vi "Controller_v6.vi"(10 "Sensors":T2) -> (0 "To Target Lossy Data":T1, 3 "Motor Command":dbl)   [LabVIEW 2018]
uses:
  Sensor Data.ctl
  Phase Calculator Feedback Cluster.ctl
  Target Lossy Data.ctl
panel:
  in  "Target Lossy Data":T1
  in  "Phase Calculator Feedback":T3
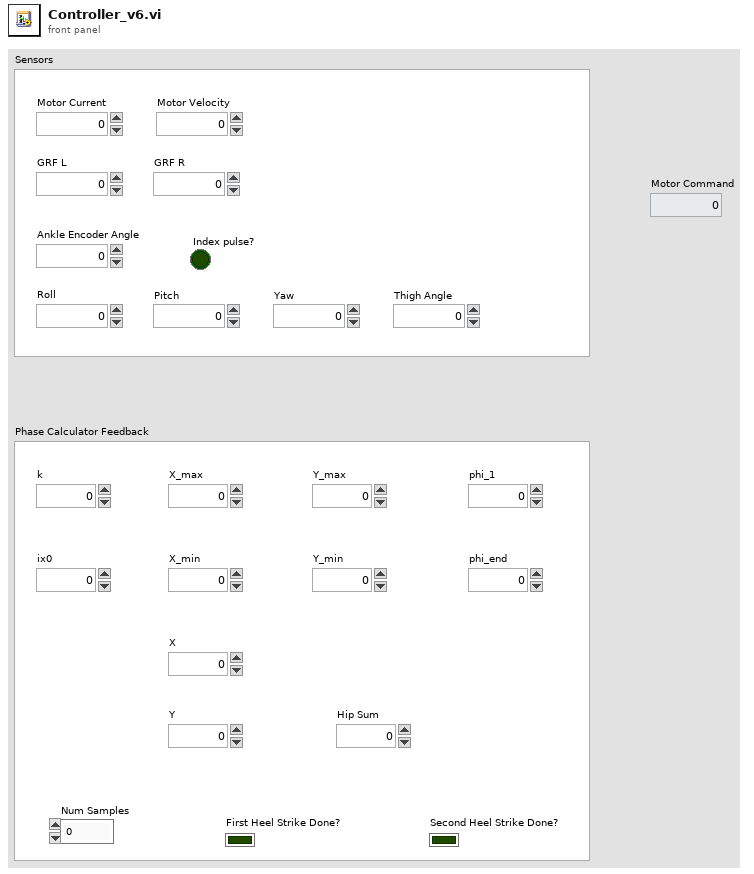
[diagram p1: front panel]
types:
  T1 = typedef "Target Lossy Data.ctl" = cluster{"Active Controller":bool, "Log Trigger":bool, "Sensors":T2, "Motor Command":dbl, "Phase Variable":dbl, "Left HS State":u32, "Left Heel Strike Pulse":bool, "Gait %":dbl, "Torque Reference":dbl, "Passive Torque":dbl, "F_th":dbl, "dF_th":dbl, "d_GRF L":dbl, "GRF L":dbl, "Transmission Ratio":dbl, "Desired Ankle Traj.":dbl, "Right HS State":u32, "Right Heel Strike Pulse":bool, "d_GRF R":dbl, "GRF R":dbl}
  T2 = typedef "Sensor Data.ctl" = cluster{"Motor Current":dbl, "Motor Velocity":dbl, "Ankle Encoder Angle":dbl, "GRF L":dbl, "GRF R":dbl, "Index pulse?":bool, "Roll":dbl, "Pitch":dbl, "Yaw":dbl, "Thigh Angle":dbl}
  T3 = typedef "Phase Calculator Feedback Cluster.ctl" = cluster{"k":dbl, "ix0":dbl, "X_max":dbl, "X_min":dbl, "Y_max":dbl, "Y_min":dbl, "Y":dbl, "Hip Sum":dbl, "Num Samples":dbl, "First Heel Strike Done?":bool, "Second Heel Strike Done?":bool, "phi_1":dbl, "phi_end":dbl, "X":dbl}
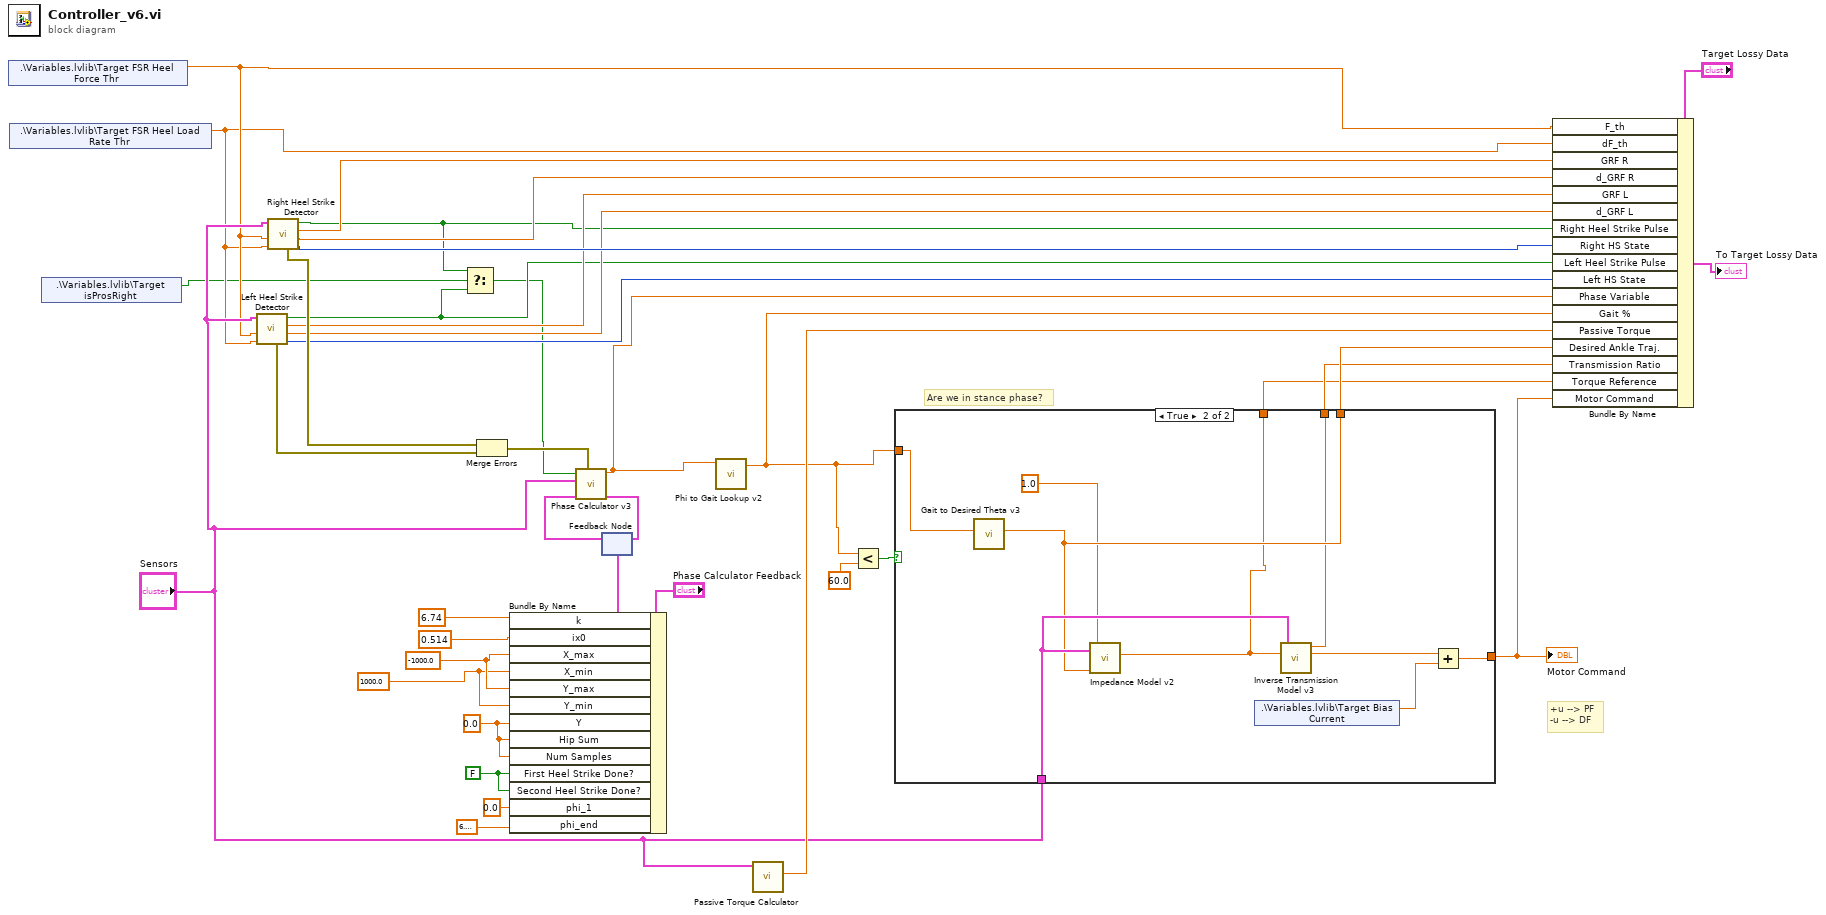
[diagram p0: block diagram]
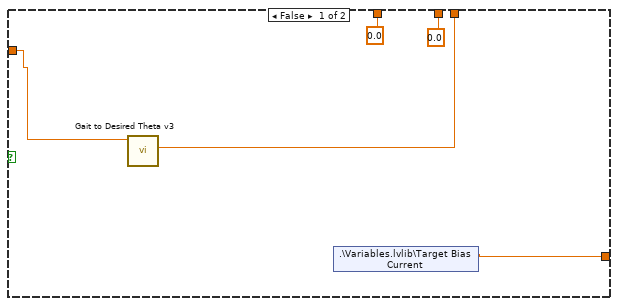
[diagram p2: hidden frame]
diagram:
  w28 = FALSE ("First Heel Strike Done?")
  w29 = 0.0 ("Y")
  w34 = 1000.0 ("X_min")
  w35 = -1000.0 ("X_max")
  # "+u --> PF\n-u --> DF"
  # "Are we in stance phase?"
  n1 = shared-variable ".\\Variables.lvlib\\Target FSR Heel Force Thr"() -> (w12:dbl)  [unwired: 1 in, 1 out]
  n2 = shared-variable ".\\Variables.lvlib\\Target FSR Heel Load Rate Thr"() -> (w11:dbl)  [unwired: 1 in, 1 out]
  n3 = shared-variable ".\\Variables.lvlib\\Target isProsRight"() -> (w6:bool)  [unwired: 1 in, 1 out]
  n4 = call "Left Heel Strike Detector.vi"("Force Rate Threshold"=w11, "Force Threshold"=w12, "Sensors"="Sensors") -> ("Heel State"=w9:i32, "d_F"=w7:dbl, "F"=w8:dbl, "Heel Strike?"=w5:bool, "error out"=w10:errorcluster)  [unwired: 4 in]
  n5 = call "Right Heel Strike Detector.vi"("Force Rate Threshold"=w11, "Force Threshold"=w12, "Sensors"="Sensors") -> ("Heel State"=w15:i32, "d_F"=w16:dbl, "F"=w17:dbl, "Heel Strike?"=w4:bool, "error out"=w14:errorcluster)  [unwired: 4 in]
  n6 = Select(t=w4, s=w6, f=w5) -> (s? t:f=w3:bool)
  n7 = Merge Errors(w14, w10) -> (w25:errorcluster)
  n8 = Bundle By Name(cluster="Phase Calculator Feedback", "k"=6.74, "ix0"=0.514, "X_max"=w35, "X_min"=w34, "Y_max"=w35, "Y_min"=w34, "Y"=w29, "Hip Sum"=w29, "Num Samples"=w29, "First Heel Strike Done?"=w28, "Second Heel Strike Done?"=w28, "phi_1"=0.0, "phi_end"=6.283185307179586) -> (w38:T3)
  n9 = feedback #1(w38) -> (w32:T3)
  n10 = call "Phase Calculator v3.vi"("error in (no error)"=w25, "Feedback In"=w32, "Sensors"="Sensors", "Heel Strike?"=w3) -> ("Feedkback Out"=w33:T3, "Phase Angle (Phi)"=w24:dbl)  [unwired: 5 in, 1 out]
  n11 = feedback-in #1(w33) -> ()
  n12 = call "Phi to Gait Lookup v2.vi"("Current Phi"=w24) -> ("Current Gait %"=w18:dbl)  [unwired: 10 in]
  n13 = call "Passive Torque Calculator.vi"("Sensors"="Sensors") -> ("Passive Torque Estimate"=w19:dbl)  [unwired: 10 in]
  n14 = Less?(x=w18, y=60.0) -> (x < y?=w27:bool)
  n15 = case shown="True" w27 {
    tunnel: [0.0 ("Tau_ref") w46] -> w20
    tunnel: "Sensors" -> [_ w53]
    tunnel: [w41 w52] -> w23
    tunnel: [0.0 ("R_tau") w51] -> w22
    tunnel: [w43 w48] -> w21
    tunnel: w18 -> [w42 w50]
    frame False {
      n16 = call "Gait to Desired Theta v3.vi"("Current Gait %"=w42) -> ("Current Desired Theta"=w41:dbl)  [unwired: 10 in]
      n17 = shared-variable ".\\Variables.lvlib\\Target Bias Current"() -> (w43:dbl)  [unwired: 1 in, 1 out]
    }
    frame True {
      n18 = call "Gait to Desired Theta v3.vi"("Current Gait %"=w50) -> ("Current Desired Theta"=w52:dbl)  [unwired: 10 in]
      n19 = call "Impedance Model v2.vi"("Theta_d"=w52, "K"=1.0, "Sensors"=w53) -> ("Tau_ref"=w46:dbl)  [unwired: 8 in]
      n20 = shared-variable ".\\Variables.lvlib\\Target Bias Current"() -> (w47:dbl)  [unwired: 1 in, 1 out]
      n21 = call "Inverse Transmission Model v3.vi"("Sensors"=w53, "Torque Reference"=w46) -> ("Motor Command"=w49:dbl, "R_tau"=w51:dbl)  [unwired: 8 in]
      n22 = Add(x=w49, y=w47) -> (x+y=w48:dbl)
    }
  }
  "Motor Command" <- w21
  n23 = Bundle By Name(cluster="Target Lossy Data", "F_th"=w12, "dF_th"=w11, "GRF R"=w17, "d_GRF R"=w16, "GRF L"=w8, "d_GRF L"=w7, "Right Heel Strike Pulse"=w4, "Right HS State"=w15, "Left Heel Strike Pulse"=w5, "Left HS State"=w9, "Phase Variable"=w24, "Gait %"=w18, "Passive Torque"=w19, "Desired Ankle Traj."=w23, "Transmission Ratio"=w22, "Torque Reference"=w20, "Motor Command"=w21) -> (→"To Target Lossy Data":T1)
